vi "global name path.vi"() -> ()   [LabVIEW 2023]
panel:
  in  "Saving Parth":path
  in  "name sample":string
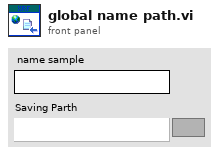
[diagram p1: front panel]
diagram:
